vi "new_try.vi"() -> ()   [LabVIEW 2010]
uses:
  <vilib>/Instr/_visa.llb/VISA Configure Serial Port (Instr).vi
panel:
  out "command to Keithley":string
  in  "output current setpoint (A)":dbl caption="setpoint" max=9999.0 format="%.4f"
  out "error out":errorcluster
  out "read buffer 2":string
  out "Bytes at Port 3":u32
  in  "RUN":bool
  in  "stop":bool
  out "actual value":string
  out "Bytes at Port":u32
  in  "Set Output Current":bool
  in  "delay (ms)":u32=500
  in  "flow control (0:none)":u16(ring) items=["None", "XON/XOFF", "RTS/CTS", "XON/XOFF & RTS/CTS", "DTR/DSR", "XON/XOFF & DTR/DSR"]
  in  "stop bits (10: 1 bit)":u16(ring)=10 items=["1.0"=10, "1.5"=15, "2.0"=20]
  in  "parity (0:none)":enum16{"None", "Odd", "Even", "Mark", "Space"}(ring)
  in  "data bits (8)":u16=8 min=5 max=8 step=1
  in  "baud rate (9600)":u32=9600
  in  "VISA resource name":refnum<visa-resource-name>="COM6"
  # "output currrent (mA)"
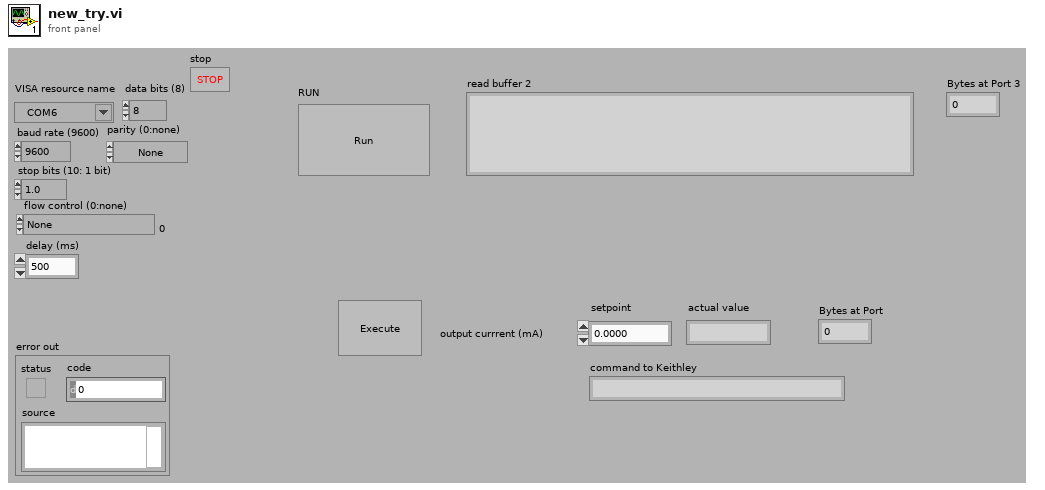
[diagram p1: front panel]
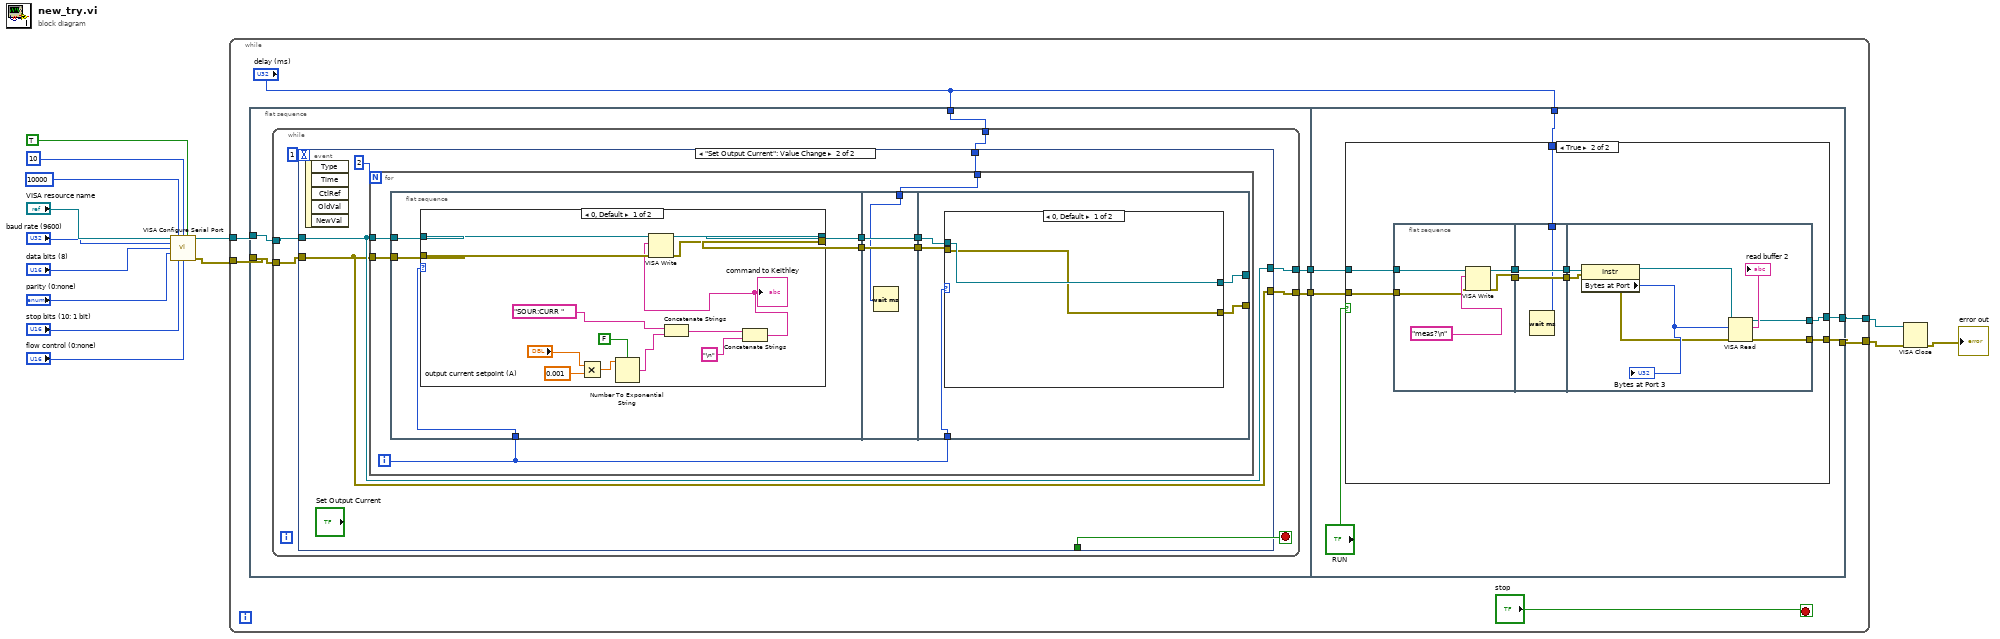
[diagram p0: block diagram]
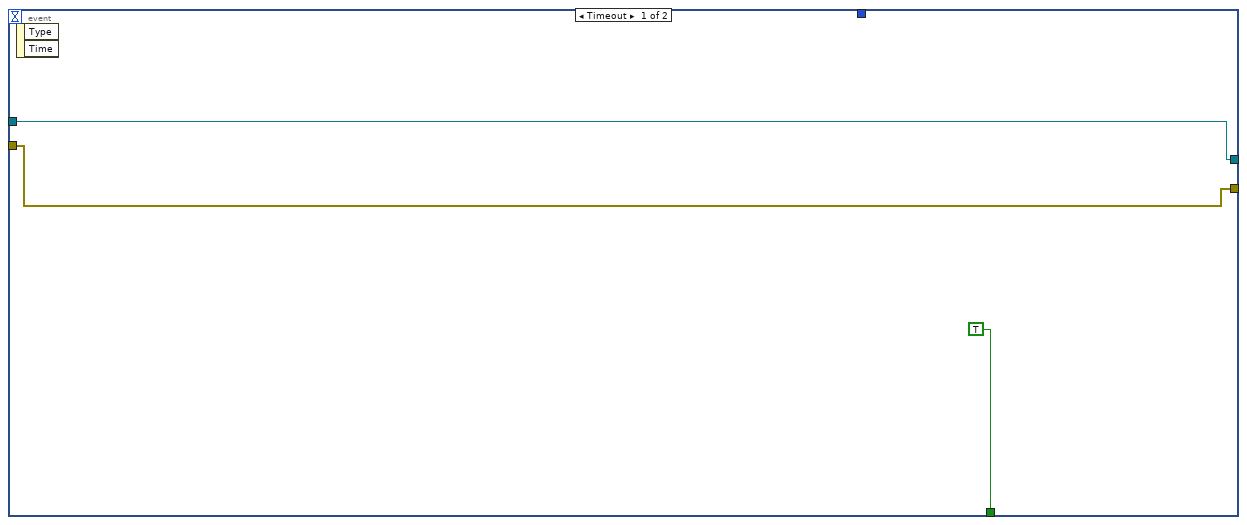
[diagram p2: hidden frame]
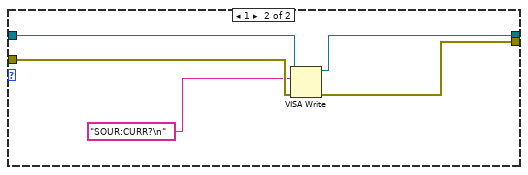
[diagram p3: hidden frame]
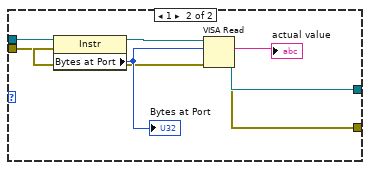
[diagram p4: hidden frame]
diagram:
  n1 = call-poly "VISA Configure Serial Port"("VISA resource name"="VISA resource name", "timeout (10sec)"=u32 10000, "termination char\n(0xA = '\\n' = LF)"=u8 10 ("termination char\n(0xA = '\\n' = LF)"), "Enable Termination\nChar (T)"=TRUE ("Enable Termination\nChar (T)"), "baud rate (9600)"="baud rate (9600)", "data bits (8)"="data bits (8)", "parity (0:none)"="parity (0:none)", "stop bits (10: 1 bit)"="stop bits (10: 1 bit)", "flow control (0:none)"="flow control (0:none)") -> ("VISA resource name out"=w5:refnum<visa-resource-name>, "error out"=w4:errorcluster)  [unwired: 5 in]
  n2 = while {
    tunnel: w5 -> [w21]
    tunnel: w4 -> [w20]
    tunnel: [w19] -> w3
    tunnel: [w18] -> w2
    stop <- "stop" stop-if-true
    n3 = flat-sequence {
      tunnel: "delay (ms)" -> [w27]
      tunnel: w21 -> [w26]
      tunnel: w20 -> [w25]
      tunnel: [w24] -> w16
      tunnel: [w23] -> w15
      tunnel: "delay (ms)" -> [w96]
      tunnel: [w95] -> w19
      tunnel: [w94] -> w18
      tunnel: w16 -> [w92]
      tunnel: w15 -> [w91]
      frame #0 {
        n4 = while {
          tunnel: w27 -> [w34]
          tunnel: w26 -> [w33]
          tunnel: w25 -> [w32]
          tunnel: [w29] -> w24
          tunnel: [w28] -> w23
          stop <- w30 stop-if-true
          n5 = event shown="[1] \"Set Output Current\": Value Change" {
            selector: _ -> [_ _]
            dyn-events: _ -> [_ _]
            timeout: 1 -> [_ _]
            tunnel: w34 -> [_ w40]
            tunnel: w33 -> [w36 w39]
            tunnel: w32 -> [w35 w38]
            tunnel: [TRUE _] -> w30
            tunnel: [w36 w39] -> w29
            tunnel: [w35 w38] -> w28
            event Timeout {
              n6 = event-data() -> ()  [unwired: 1 in, 2 out]
            }
            event "Set Output Current": Value Change {
              n7 = event-data() -> ()  [unwired: 1 in, 5 out]
              n8 = for {
                N: 2 -> [_]
                tunnel: w40 -> [w44]
                tunnel: w39 -> [w43]
                tunnel: w38 -> [w42]
                i -> [w47]
                n9 = flat-sequence {
                  tunnel: [w54] -> w49
                  tunnel: w47 -> [w53]
                  tunnel: [w52] -> w46
                  tunnel: w43 -> [w51]
                  tunnel: w42 -> [w50]
                  tunnel: w49 -> [w75]
                  tunnel: [w75] -> w48
                  tunnel: w46 -> [w74]
                  tunnel: [w74] -> w45
                  tunnel: w44 -> [w73]
                  tunnel: w48 -> [w80]
                  tunnel: w47 -> [w79]
                  tunnel: w45 -> [w78]
                  tunnel: [w77] -> _
                  tunnel: [w76] -> _
                  frame #0 {
                    n10 = case shown="0, Default" w53 {
                      tunnel: [w67 w69] -> w54
                      tunnel: [w66 w68] -> w52
                      tunnel: w51 -> [w65 w71]
                      tunnel: w50 -> [w64 w72]
                      frame 0, Default {
                        n11 = Multiply(x="output current setpoint (A)", y=0.001) -> (x*y=w56:dbl)
                        n12 = Number To Exponential String(number=w56, 1:FALSE ("use system decimal point (T)")) -> (E-format string=w62:string)  [unwired: 2 in]
                        n13 = Concatenate Strings("SOUR:CURR " ("string"), w62) -> (w60:string)
                        n14 = Concatenate Strings(w60, "\n" ("string")) -> (w59:string)
                        "command to Keithley" <- w59
                        n15 = VISA Write(VISA resource name=w65, write buffer=w59, error in (no error)=w64) -> (VISA resource name out=w67:refnum<visa-resource-name>, error out=w66:errorcluster)  [unwired: 1 out]
                      }
                      frame 1 {
                        n16 = VISA Write(VISA resource name=w71, write buffer="SOUR:CURR?\n" ("string"), error in (no error)=w72) -> (VISA resource name out=w69:refnum<visa-resource-name>, error out=w68:errorcluster)  [unwired: 1 out]
                      }
                    }
                  }
                  frame #1 {
                    n17 = Wait (ms)(milliseconds to wait=w73) -> ()  [unwired: 1 out]
                  }
                  frame #2 {
                    n18 = case shown="0, Default" w79 {
                      tunnel: w80 -> [w82 w86]
                      tunnel: w78 -> [w81 w85]
                      tunnel: [w82 w84] -> w77
                      tunnel: [w81 w83] -> w76
                      frame 0, Default {
                      }
                      frame 1 {
                        n19 = property class="Instr"(reference=w86, error in=w85) -> (reference out=w88:refnum<visa-resource-name>, error out=w87:errorcluster, "Bytes at Port"=w90:u32)
                        "Bytes at Port" <- w90
                        n20 = VISA Read(VISA resource name=w88, byte count=w90, error in (no error)=w87) -> (VISA resource name out=w84:refnum<visa-resource-name>, read buffer=→"actual value":string, error out=w83:errorcluster)  [unwired: 1 out]
                      }
                    }
                  }
                }
              }
            }
          }
        }
      }
      frame #1 {
        n21 = case shown="True" "RUN" {
          tunnel: w96 -> [_ w103]
          tunnel: [w98 w102] -> w95
          tunnel: [w97 w101] -> w94
          tunnel: w92 -> [w98 w100]
          tunnel: w91 -> [w97 w99]
          frame False {
          }
          frame True {
            n22 = flat-sequence {
              tunnel: [w112] -> w107
              tunnel: [w111] -> w106
              tunnel: w100 -> [w109]
              tunnel: w99 -> [w108]
              tunnel: w107 -> [w115]
              tunnel: [w115] -> w105
              tunnel: w106 -> [w114]
              tunnel: [w114] -> w104
              tunnel: w103 -> [w113]
              tunnel: w105 -> [w119]
              tunnel: w104 -> [w118]
              tunnel: [w117] -> w101
              tunnel: [w116] -> w102
              frame #0 {
                n23 = VISA Write(VISA resource name=w109, write buffer="meas?\n" ("write buffer 2"), error in (no error)=w108) -> (VISA resource name out=w112:refnum<visa-resource-name>, error out=w111:errorcluster)  [unwired: 1 out]
              }
              frame #1 {
                n24 = Wait (ms)(milliseconds to wait=w113) -> ()  [unwired: 1 out]
              }
              frame #2 {
                n25 = property class="Instr"(reference=w119, error in=w118) -> (reference out=w121:refnum<visa-resource-name>, error out=w120:errorcluster, "Bytes at Port"=w123:u32)
                "Bytes at Port 3" <- w123
                n26 = VISA Read(VISA resource name=w121, byte count=w123, error in (no error)=w120) -> (VISA resource name out=w116:refnum<visa-resource-name>, read buffer=→"read buffer 2":string, error out=w117:errorcluster)  [unwired: 1 out]
              }
            }
          }
        }
      }
    }
  }
  n27 = VISA Close(VISA resource name=w3, error in (no error)=w2) -> (error out=→"error out":errorcluster)
